vi "Read Pressure Sensor Settings.vi"(8 "error in (no error)":errorcluster, 11 "Boot Loader in":refnum<class "Boot Loader.lvclass">) -> (0 "error out":errorcluster, 2 "Pressure Sensor Settings":T1 {"Offset" format="%_6f"; "PSI per Volt" format="%_6f"}, 3 "Boot Loader out":refnum<class "Boot Loader.lvclass">)   [LabVIEW 2015, in "Boot Loader.lvclass"]
uses:
  Boot Loader.lvclass
  Typedefs/Pressure Sensor Settings.ctl
  Settings/Settings.lvclass
  Typedefs/FAMT Typedefs.lvlib
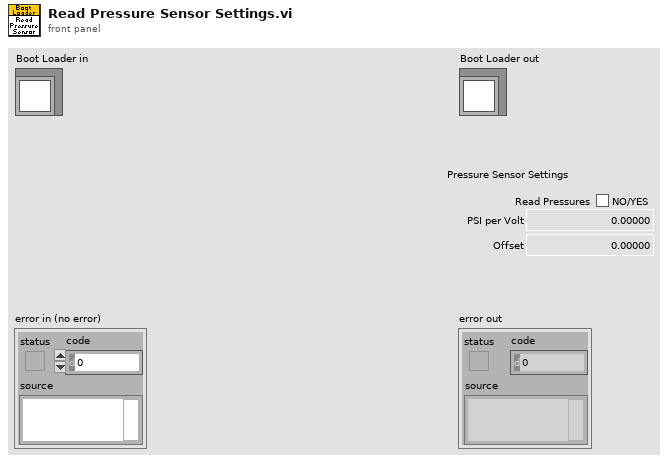
[diagram p1: front panel]
types:
  T1 = typedef "FAMT Typedefs.lvlib/Pressure Sensor Settings.ctl" = cluster{"Read Pressures":bool, "PSI per Volt":dbl, "Offset":dbl}
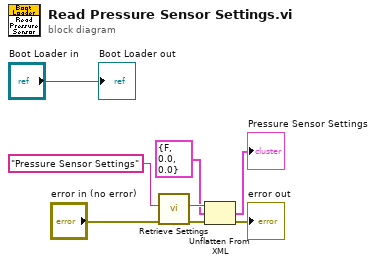
[diagram p0: block diagram]
diagram:
  n1 = call "Retrieve Settings.vi"("error in (no error)"="error in (no error)", "configName"="Pressure Sensor Settings") -> ("error out"=w7:errorcluster, "xmlConfig"=w6:string)  [unwired: 7 in, 1 out]
  n2 = Unflatten From XML(xml string=w6, type=T1 {"Read Pressures"=FALSE, "PSI per Volt"=0.0, "Offset"=0.0} ("Pressure Sensor Settings 2"), error in (no error)=w7) -> (value=→"Pressure Sensor Settings":T1, error out=→"error out":errorcluster)
  "Boot Loader out" <- "Boot Loader in"
